vi "Digital Read Pulse Width.vi"(5 "Incoming Pulse Polarity (Active High)":T2=enum."Active High", 6 "Timeout  (250 mS)":u32=250, 7 "Stimulus Pulse (Active High)":T1=enum."Active High", 8 "Error In":errorcluster={"status"=FALSE, "code"=1073676294, "source"="VISA Read in LVH-LINX.lvlib:Device.lvlib:Serial Read.vi->LVH-LINX.lvlib:Device.lvlib:Wait For Packet.vi->LVH-LINX.lvlib:Device.lvlib:Send Command.vi->LVH-LINX.lvlib:Device.lvlib:Digital Read Pulse Width.vi->Untitled 5"}, 9 "DO Channel (0)":u8, 10 "DI Channel (0)":u8=8, 11 "LINX Device Config":T3={"Interface"=enum."Serial", "COM Port"="COM5", "TCP Configuration"={"IP Address"="", "Port"=0}, "Device Family"=enum."Digilent", "Device ID"=1, "Device Name"="chipKIT uC32", "TCP Ref"=refnum}) -> (0 "Error Out":errorcluster={"status"=FALSE, "code"=1073676294, "source"="VISA Read in LVH-LINX.lvlib:Device.lvlib:Serial Read.vi->LVH-LINX.lvlib:Device.lvlib:Wait For Packet.vi->LVH-LINX.lvlib:Device.lvlib:Send Command.vi->LVH-LINX.lvlib:Device.lvlib:Digital Read Pulse Width.vi->Untitled 5"}, 2 "Pulse Width (uS)":u32, 3 "LINX Device Config":T3={"Interface"=enum."Serial", "COM Port"="COM5", "TCP Configuration"={"IP Address"="", "Port"=0}, "Device Family"=enum."Digilent", "Device ID"=1, "Device Name"="chipKIT uC32", "TCP Ref"=refnum})   [LabVIEW 2013, in "LVH-LINX.lvlib" / "Device.lvlib"]
uses:
  <vilib>/LabVIEW Hacker/LINX/Private/Device/Device.lvlib
  <vilib>/LabVIEW Hacker/LINX/Private/Device/Type Defs/LINX Device Config.ctl
  <vilib>/LabVIEW Hacker/LINX/Private/Type Defs/Interface.ctl
  <vilib>/LabVIEW Hacker/LINX/Private/Device/Type Defs/TCP Config.ctl
  <vilib>/LabVIEW Hacker/LINX/Private/Type Defs/Device Family.ctl
  <vilib>/LabVIEW Hacker/LINX/Private/Device/Type Defs/Pulse Polarity.ctl
  <vilib>/LabVIEW Hacker/LINX/Private/Device/Type Defs/Stimulus Pulse.ctl
  <vilib>/LabVIEW Hacker/LINX/Private/Type Defs/Error Type.ctl
  <vilib>/LabVIEW Hacker/LINX/LVH-LINX.lvlib
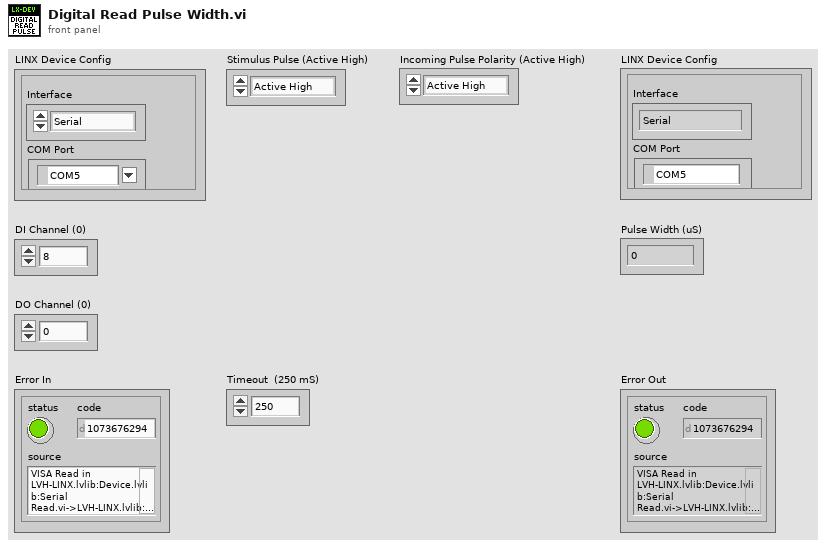
[diagram p1: front panel]
types:
  T1 = typedef "LVH-LINX.lvlib/Device.lvlib/Stimulus Pulse.ctl" = enum16{"None", "Active Low", "Active High"}
  T2 = typedef "LVH-LINX.lvlib/Device.lvlib/Pulse Polarity.ctl" = enum8{"Active Low", "Active High"}
  T3 = typedef "LVH-LINX.lvlib/Device.lvlib/LINX Device Config.ctl" = cluster{"Interface":T4, "COM Port":refnum<visa-resource-name>, "TCP Configuration":T5, "Device Family":T6, "Device ID":u8, "Device Name":string, "TCP Ref":refnum<k5>}
  T4 = typedef "LVH-LINX.lvlib/Interface.ctl" = enum16{"Serial", "TCP"}
  T5 = typedef "LVH-LINX.lvlib/Device.lvlib/TCP Config.ctl" = cluster{"IP Address":string, "Port":u16}
  T6 = typedef "LVH-LINX.lvlib/Device Family.ctl" = enum8{"National Instruments", "Digilent", "Arduino"}
  T7 = typedef "LVH-LINX.lvlib/Error Type.ctl" = enum16{"Unknown", "Timeout", "Corrupt Return Packet", "Unable To Connect", "Command Not Supported", "Channel DNE", "Invalid COM Config"}
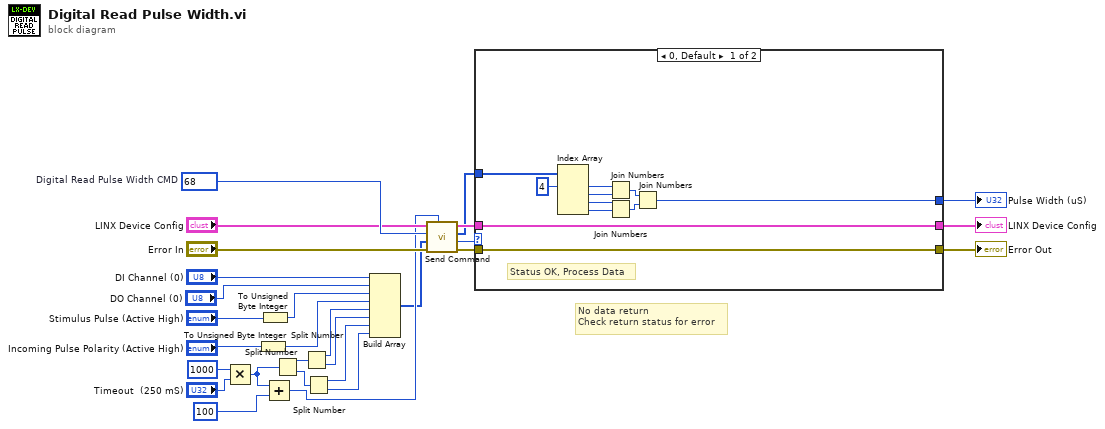
[diagram p0: block diagram]
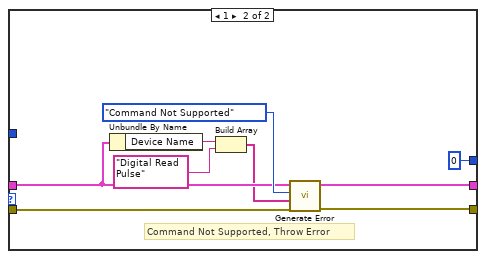
[diagram p2: hidden frame]
diagram:
  w27 = u16 68  # Digital Read Pulse Width CMD
  # "No data return\nCheck return status for error"
  n1 = Multiply(x=u32 1000 ("y"), y="Timeout  (250 mS)") -> (x*y=w5:u32)
  n2 = To Unsigned Byte Integer(number="Incoming Pulse Polarity (Active High)") -> (unsigned 8bit integer=w19:u8)
  n3 = To Unsigned Byte Integer(number="Stimulus Pulse (Active High)") -> (unsigned 8bit integer=w21:u8)
  n4 = Add(x=w5, y=u32 100) -> (x+y=w17:u32)
  n5 = Split Number(x=w5) -> (hi(x)=w16:u16, lo(x)=w15:u16)
  n6 = Split Number(x=w16) -> (hi(x)=w14:u8, lo(x)=w13:u8)
  n7 = Split Number(x=w15) -> (hi(x)=w12:u8, lo(x)=w11:u8)
  n8 = Build Array("DI Channel (0)", "DO Channel (0)", w21, w19, w14, w13, w12, w11) -> (w10:u8[])
  n9 = call <vilib>:"Send Command.vi"("Timeout (100 ms)"=w17, "Error In"="Error In", "ARGS"=w10, "CMD"=w27, "LINX Device Config"="LINX Device Config") -> ("Error Out"=w22:errorcluster, "Status"=w9:u8, "Response"=w8:u8[], "LINX Device Config"=w24:T3)  [unwired: 3 in]
  n10 = case shown="0, Default" w9 {
    tunnel: [w39 w46] -> w25
    tunnel: w24 -> [w39 w42]
    tunnel: [w38 w47] -> w23
    tunnel: w22 -> [w38 w48]
    tunnel: w8 -> [w37 _]
    tunnel: [w29 u32 0] -> w7
    frame 0, Default {
      # "Status OK, Process Data"
      n11 = Index Array(array=w37, index #1=4 ("index")) -> (element #1=w35:u8, element #2=w34:u8, element #3=w33:u8, element #4=w32:u8)  [unwired: 3 in]
      n12 = Join Numbers(hi=w35, lo=w34) -> ((hi.lo)=w31:u16)
      n13 = Join Numbers(hi=w33, lo=w32) -> ((hi.lo)=w30:u16)
      n14 = Join Numbers(hi=w31, lo=w30) -> ((hi.lo)=w29:u32)
    }
    frame 1 {
      # "Command Not Supported, Throw Error"
      n15 = Unbundle By Name(w42) -> ("Device Name"=w44:string)
      n16 = Build Array(w44, "Digital Read Pulse") -> (w41:string[])
      n17 = call <vilib>:"Generate Error.vi"("Error In"=w48, "Arguments"=w41, "Error Type"=Error_Type."Command Not Supported", "LINX Device Config"=w42) -> ("Error Out"=w47:errorcluster, "LINX Device Config"=w46:T3)  [unwired: 6 in]
    }
  }
  "Error Out" <- w23
  "LINX Device Config" <- w25
  "Pulse Width (uS)" <- w7
